vi "LaserCal-Process Data (I-O).vi"(0 "Time Graph":refnum<vi>, 5 "I-O":refnum<vi>, 7 "Power (W)":dbl, 9 "I-O Data in":T1, 11 "error in (no error)":errorcluster, 12 "Seq Index":i32, 13 "Time (s)":dbl) -> (10 "I-O Data out":T1, 15 "error out":errorcluster)   [LabVIEW 2015]
uses:
  Typedefs/LaserCal-Data (I-O).ctl
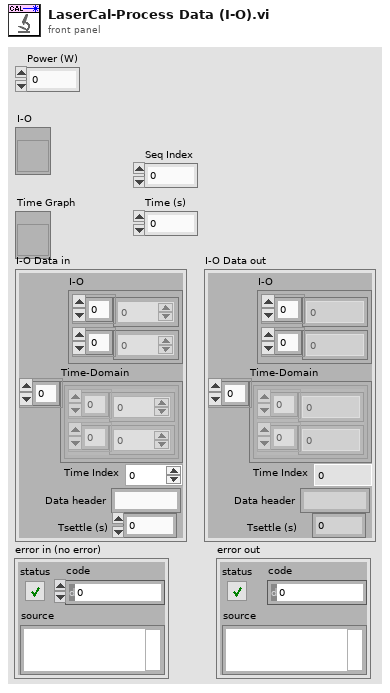
[diagram p1: front panel]
types:
  T1 = typedef "LaserCal-Data (I-O).ctl" = cluster{"I-O":cluster{dbl[], dbl[]}, "Time-Domain":cluster{dbl[], dbl[]}[], "Time Index":i32, "Data header":string, "Tsettle (s)":dbl}
  T2 = typedef "LVRangeTypeDef.ctl" = cluster{"Minimum":dbl, "Maximum":dbl, "Increment":dbl, "Minor Increment":dbl, "Start":dbl}
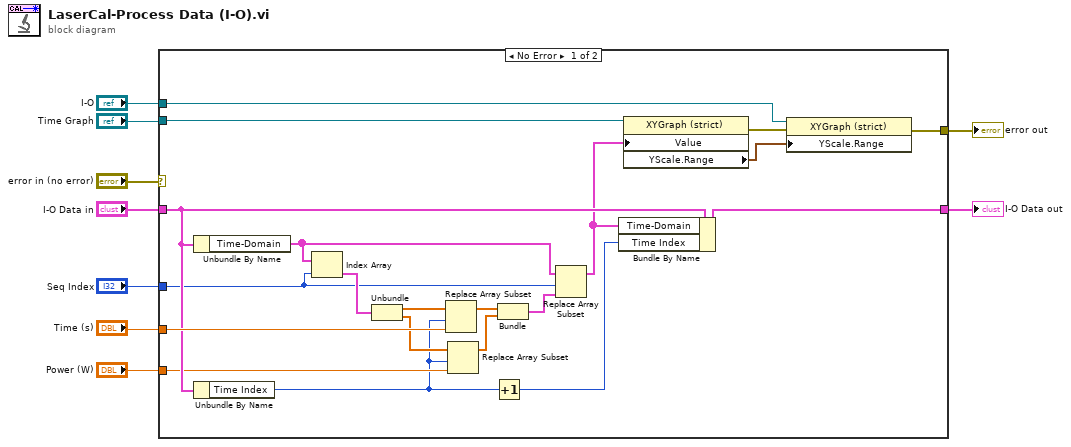
[diagram p0: block diagram]
diagram:
  n1 = case shown="No Error" "error in (no error)" {
    selector: "error in (no error)" -> [_ w31]
    tunnel: [w10 w31] -> w2
    tunnel: "I-O Data in" -> [w27 w30]
    tunnel: [w18 w30] -> w4
    tunnel: "Seq Index" -> [w21 _]
    tunnel: "Time (s)" -> [w28 _]
    tunnel: "Power (W)" -> [w26 _]
    tunnel: "Time Graph" -> [w15 _]
    tunnel: "I-O" -> [w12 _]
    frame No Error {
      n2 = Unbundle By Name(w27) -> ("Time-Domain"=w19:cluster{dbl[], dbl[]}[])
      n3 = Unbundle By Name(w27) -> ("Time Index"=w17:i32)
      n4 = Index Array(array=w19, index=w21) -> (element=w22:cluster{dbl[], dbl[]})
      n5 = Unbundle(w22) -> (w29:dbl[], w25:dbl[])
      n6 = Replace Array Subset(array=w29, new element=w28, index=w17) -> (w24:dbl[])
      n7 = Replace Array Subset(array=w25, new element=w26, index=w17) -> (w23:dbl[])
      n8 = Increment(x=w17) -> (x+1=w16:i32)
      n9 = Bundle(w24, w23) -> (w20:cluster{dbl[], dbl[]})  [unwired: 1 in]
      n10 = Replace Array Subset(array=w19, new element=w20, index=w21) -> (w14:cluster{dbl[], dbl[]}[])
      n11 = Bundle By Name(cluster=w27, "Time-Domain"=w14, "Time Index"=w16) -> (w18:T1)
      n12 = property class="XYGraph (strict)"(reference=w15, "Value"=w14) -> (error out=w13:errorcluster, "YScale.Range"=w11:T2)  [unwired: 1 in, 1 out]
      n13 = property class="XYGraph (strict)"(reference=w12, error in=w13, "YScale.Range"=w11) -> (error out=w10:errorcluster)  [unwired: 1 out]
    }
    frame Error {
    }
  }
  "I-O Data out" <- w4
  "error out" <- w2
